vi "DriveStraight.vi"(7 "Sensitivity":dbl=0.02 format="%#_13g", 8 "Range":dbl, 9 "Motor Speed":dbl, 10 "Target":dbl, 11 "Yaw":dbl) -> (0 "Right":dbl, 3 "Left":dbl)   [LabVIEW 2015]
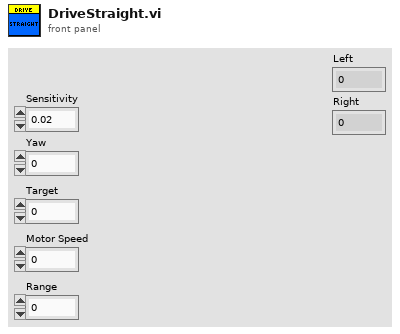
[diagram p1: front panel]
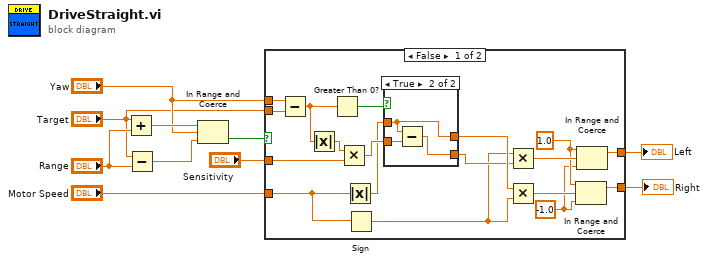
[diagram p0: block diagram]
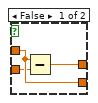
[diagram p2: hidden frame]
diagram:
  n1 = Add(x="Target", y="Range") -> (x+y=w10:dbl)
  n2 = Subtract(x="Target", y="Range") -> (x-y=w9:dbl)
  n3 = In Range and Coerce(upper limit=w10, x="Yaw", lower limit=w9) -> (In Range?=w7:bool)  [unwired: 1 out]
  n4 = case shown="False" w7 {
    tunnel: "Motor Speed" -> [w23 w35]
    tunnel: [w13 w35] -> w2
    tunnel: "Yaw" -> [w28 _]
    tunnel: "Target" -> [w27 _]
    tunnel: [w14 w35] -> w3
    tunnel: "Sensitivity" -> [w19 _]
    frame False {
      w16 = 1.0 ("upper limit")
      w15 = -1.0 ("lower limit")
      n5 = Subtract(x=w28, y=w27) -> (x-y=w11:dbl)
      n6 = Absolute Value(x=w11) -> (abs(x)=w12:dbl)
      n7 = Greater Than 0?(x=w11) -> (x > 0?=w26:bool)
      n8 = Multiply(x=w12, y=w19) -> (x*y=w25:dbl)
      n9 = Absolute Value(x=w23) -> (abs(x)=w24:dbl)
      n10 = Sign(1:w23) -> (0:w20:dbl)
      n11 = case shown="True" w26 {
        tunnel: w24 -> [w31 w33]
        tunnel: [w30 w33] -> w22
        tunnel: [w31 w34] -> w21
        tunnel: w25 -> [w29 w32]
        frame False {
          n12 = Subtract(x=w31, y=w29) -> (x-y=w30:dbl)
        }
        frame True {
          n13 = Subtract(x=w33, y=w32) -> (x-y=w34:dbl)
        }
      }
      n14 = Multiply(x=w20, y=w21) -> (x*y=w18:dbl)
      n15 = Multiply(x=w22, y=w20) -> (x*y=w17:dbl)
      n16 = In Range and Coerce(upper limit=w16, x=w17, lower limit=w15) -> (coerced(x)=w13:dbl)  [unwired: 1 out]
      n17 = In Range and Coerce(upper limit=w16, x=w18, lower limit=w15) -> (coerced(x)=w14:dbl)  [unwired: 1 out]
    }
    frame True {
    }
  }
  "Left" <- w3
  "Right" <- w2
